vi "Remove Items.vi"(8 "error in (no error)":errorcluster, 10 "Methods":string, 11 "LUnit Test Suite In":refnum<class "LUnit Test Suite.lvclass">) -> (0 "error out":errorcluster, 3 "LUnit Test Suite Out":refnum<class "LUnit Test Suite.lvclass">)   [LabVIEW 2020, in "LUnit Test Suite.lvclass"]
uses:
  LUnit Test Suite.lvclass
  C:/git/astemes-lunit/source/Core/Runnable/Runnable.lvclass
  LUnit Test Suite.lvclass/LUnit Test Suite.ctl
  Core/Runnable/Runnable.lvclass
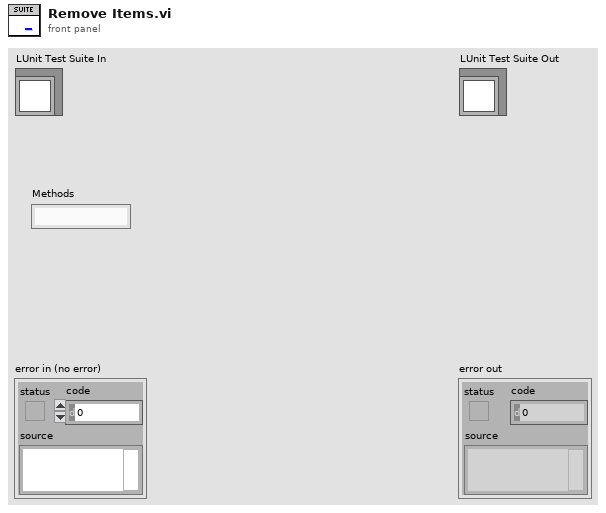
[diagram p1: front panel]
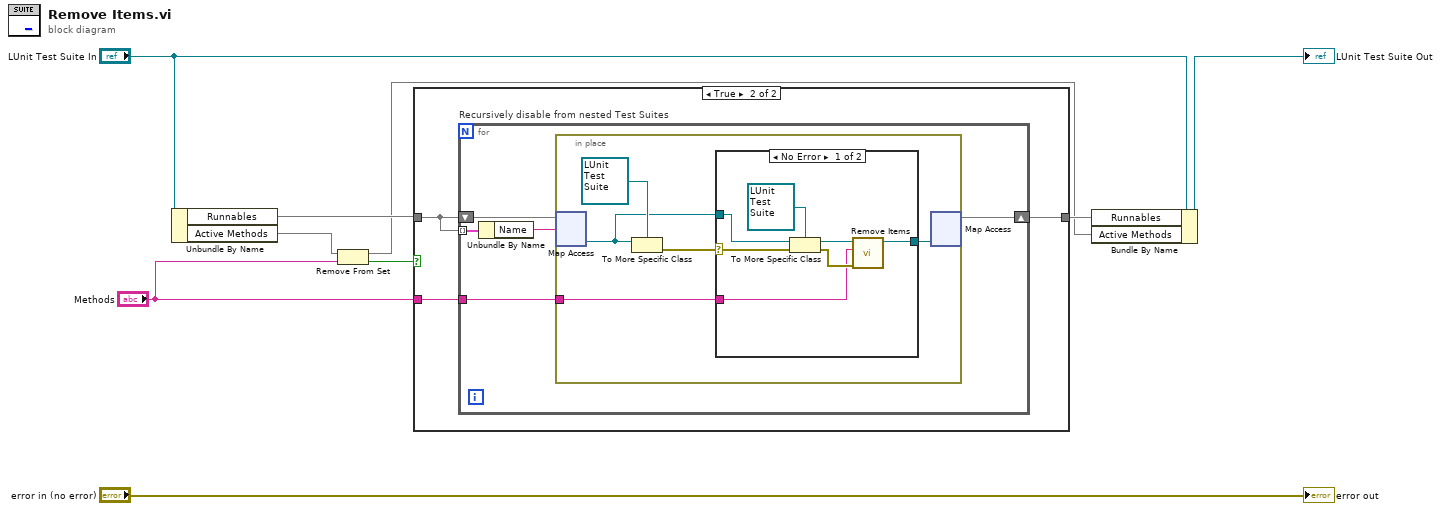
[diagram p0: block diagram]
diagram:
  n1 = Unbundle By Name("LUnit Test Suite In") -> ("Runnables"=w7:map{string, refnum<class "Runnable.lvclass">}, "Active Methods"=w4:set{string})
  n2 = Remove From Set(10:"Methods", 11:w4) -> (2:w2:bool, 3:w1:set{string})
  n3 = case shown="True" w2 {
    tunnel: w7 -> [w10 w13]
    tunnel: [w10 w12] -> w5
    tunnel: "Methods" -> [_ w11]
    frame False {
    }
    frame True {
      n4 = for "Recursively disable from nested Test Suites" {
        shift-right: [w17] -> w12
        shift-left: w13 -> [w18]
        tunnel: w13 -> [w15] mode=indexing
        tunnel: w11 -> [w16]
        n5 = Unbundle By Name(w15) -> ("Name"=w14:string)
        n6 = in-place {
          in-place-border: w16 -> [w19]
          n7 = in-place-map #1(w18, w14) -> (w21:refnum<class "Runnable.lvclass">)  [unwired: 1 in, 1 out]
          n8 = To More Specific Class(target class=refnum<class "LUnit Test Suite.lvclass"> refnum ("LUnit Test Suite V2.lvclass"), reference=w21) -> (error out=w22:errorcluster)  [unwired: 1 in, 1 out]
          n9 = case shown="No Error" w22 {
            selector: w22 -> [w28 _]
            tunnel: w21 -> [w29 w31]
            tunnel: [w25 w31] -> w20
            tunnel: w19 -> [w24 _]
            frame No Error {
              n10 = To More Specific Class(target class=refnum<class "LUnit Test Suite.lvclass"> refnum ("LUnit Test Suite V2.lvclass"), reference=w29, error in=w28) -> (specific class reference=w27:refnum<class "LUnit Test Suite.lvclass">, error out=w26:errorcluster)
              n11 = call "Remove Items.vi"("error in (no error)"=w26, "Methods"=w24, "LUnit Test Suite In"=w27) -> ("LUnit Test Suite Out"=w25:refnum<class "LUnit Test Suite.lvclass">)  [unwired: 7 in, 1 out]
            }
            frame Error {
            }
          }
          n12 = in-place-map #1(w20) -> (w17:map{string, refnum<class "Runnable.lvclass">})  [unwired: 1 in, 2 out]
        }
      }
    }
  }
  n13 = Bundle By Name(cluster="LUnit Test Suite In", "Runnables"=w5, "Active Methods"=w1) -> (→"LUnit Test Suite Out":refnum<class "LUnit Test Suite.lvclass">)
  "error out" <- "error in (no error)"
